vi "Initialize Attributes.vi"(8 "error in (no error)":errorcluster, 10 "Attribute Data":variant, 11 "BNT_DAQmx-MCSV-AIAvg in":refnum<class "BNT_DAQmx-MCSV-AIAvg.lvclass">) -> (0 "error out":errorcluster, 2 "MandatoryParameters":cluster{"Parameter":string, "found?":bool}[](array[cluster]), 3 "BNT_DAQmx-MCSV-AIAvg out":refnum<class "BNT_DAQmx-MCSV-AIAvg.lvclass">)   [LabVIEW 2017, in "BNT_DAQmx.lvlib" / "BNT_DAQmx-MCSV-AIAvg.lvclass"]
doc: "Initialize object attribute.\n\nUnique resources should be allocated elsewhere!"
uses:
  BNT_DAQmx-MCSV-AIAvg.lvclass
  BNT_DAQmx-MCSV-AIAvg.lvclass/BNT_DAQmx-MCSV-AIAvg.ctl
  BNT_DAQmx-MCSV/BNT_DAQmx-MCSV.lvclass
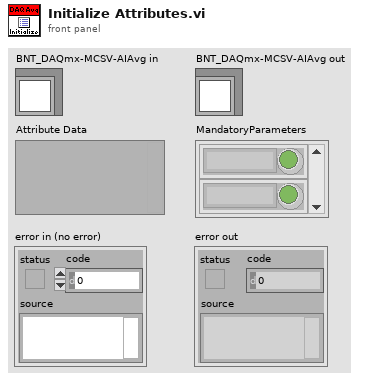
[diagram p1: front panel]
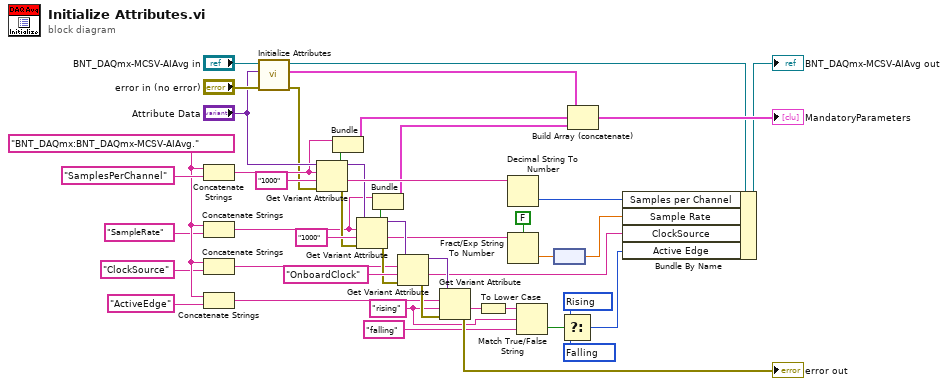
[diagram p0: block diagram]
diagram:
  w15 = 10171 items=["Rising"=10280, "Falling"=10171] ("Active Edge")
  w14 = 10280 items=["Rising"=10280, "Falling"=10171] ("Active Edge")
  w3 = "rising" ("string")
  w22 = "BNT_DAQmx:BNT_DAQmx-MCSV-AIAvg."
  n1 = Concatenate Strings(w22, "SamplesPerChannel" ("string")) -> (w39:string)
  n2 = Concatenate Strings(w22, "SampleRate" ("string")) -> (w18:string)
  n3 = Concatenate Strings(w22, "ClockSource" ("string")) -> (w17:string)
  n4 = Concatenate Strings(w22, "ActiveEdge" ("string")) -> (w16:string)
  n5 = call-parent "Initialize Attributes.vi"("error in (no error)"="error in (no error)", "Attribute Data"="Attribute Data", "BNT_DAQmx-MCSV in"="BNT_DAQmx-MCSV-AIAvg in") -> ("error out"=w7:errorcluster, "MandatoryParameters"=w46:cluster{"Parameter":string, "found?":bool}[], "BNT_DAQmx-MCSV out"=w36:refnum<class "BNT_DAQmx-MCSV-AIAvg.lvclass">)  [unwired: 6 in]
  n6 = Get Variant Attribute(Variant="Attribute Data", name=w39, default value (empty Variant)="1000" ("string"), error in=w7) -> (duplicate Variant=w29:variant, found=w40:bool, value=w34:string, error out=w24:errorcluster)
  n7 = Bundle(w39, w40) -> (w37:cluster{string, bool})  [unwired: 1 in]
  n8 = Get Variant Attribute(Variant=w29, name=w18, default value (empty Variant)="1000" ("string"), error in=w24) -> (duplicate Variant=w28:variant, found=w32:bool, value=w11:string, error out=w25:errorcluster)
  n9 = Bundle(w18, w32) -> (w23:cluster{string, bool})  [unwired: 1 in]
  n10 = Get Variant Attribute(Variant=w28, name=w17, default value (empty Variant)="OnboardClock" ("string"), error in=w25) -> (duplicate Variant=w27:variant, value=w12:string, error out=w26:errorcluster)  [unwired: 1 out]
  n11 = Get Variant Attribute(Variant=w27, name=w16, default value (empty Variant)=w3, error in=w26) -> (value=w5:string, error out=→"error out":errorcluster)  [unwired: 2 out]
  n12 = To Lower Case(string=w5) -> (all lower case string=w4:string)
  n13 = Decimal String To Number(string=w34) -> (number=w33:i32)  [unwired: 2 in, 1 out]
  n14 = Fract/Exp String To Number(use system decimal point (T)=FALSE, string=w11) -> (number=w9:dbl)  [unwired: 2 in, 1 out]
  n15 = Match True/False String(2:"falling" ("string"), 3:w3, 4:w4) -> (0:w1:bool)  [unwired: 1 out]
  n16 = node(w9) -> (w8:dbl[unit])
  n17 = Select(t=w14, s=w1, f=w15) -> (s? t:f=w13:i32)
  n18 = Build Array (concatenate)(w46, w37, w23) -> (→"MandatoryParameters":cluster{"Parameter":string, "found?":bool}[])
  n19 = Bundle By Name(cluster=w36, "Samples per Channel"=w33, "Sample Rate"=w8, "ClockSource"=w12, "Active Edge"=w13) -> (→"BNT_DAQmx-MCSV-AIAvg out":refnum<class "BNT_DAQmx-MCSV-AIAvg.lvclass">)
